vi ".LVLIBP CD XML Updater.vi"(5 "Files Generated by Build":path[](array[path]), 6 "Top Level/Always Included VIs":path[](array[path]), 7 "Destination Path":path, 8 "error in (no error)":errorcluster, 9 "Target Name":string, 10 "Build Specification Name":string, 11 "Project Path":path) -> (0 "error out":errorcluster)   [LabVIEW 2018]
doc: "This VI is called after each run of a build specification. The VI will copy the generated LLB (Engine or System Explorer) into the VeriStand Custom Device folder (...\\Documents\\National Instruments\\NI VeriStand 2013...)."
uses:
  .LVLIBP CD XML Updater/Project XML Editor/Project XML Editor.lvclass/Project XML Editor.ctl
  <vilib>/xml/Close Reference(Node).vi
  .LVLIBP CD XML Updater/.LVLIBP CD XML Updater.lvlib
  .LVLIBP CD XML Updater/LVLIBP Parser/LVLIBP Parser.lvclass
  .LVLIBP CD XML Updater/Project XML Editor/Project XML Editor.lvclass
  <vilib>/xml/NI_XML.lvlib
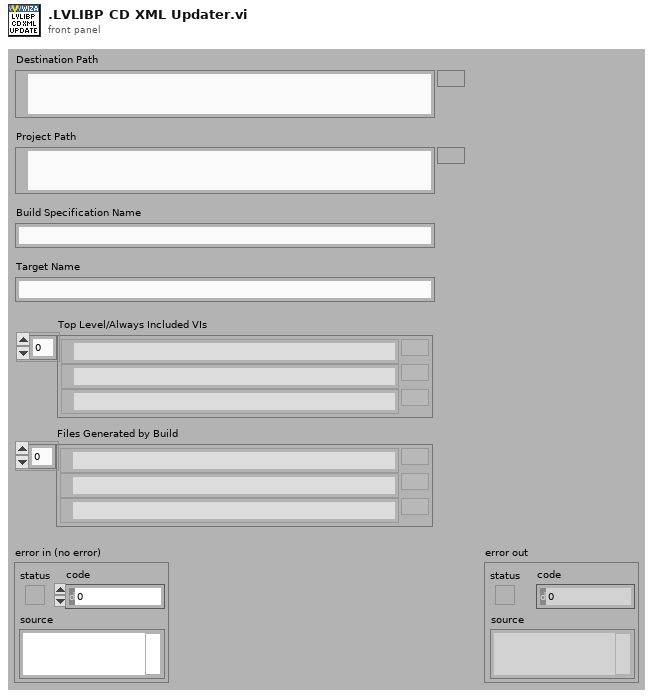
[diagram p1: front panel]
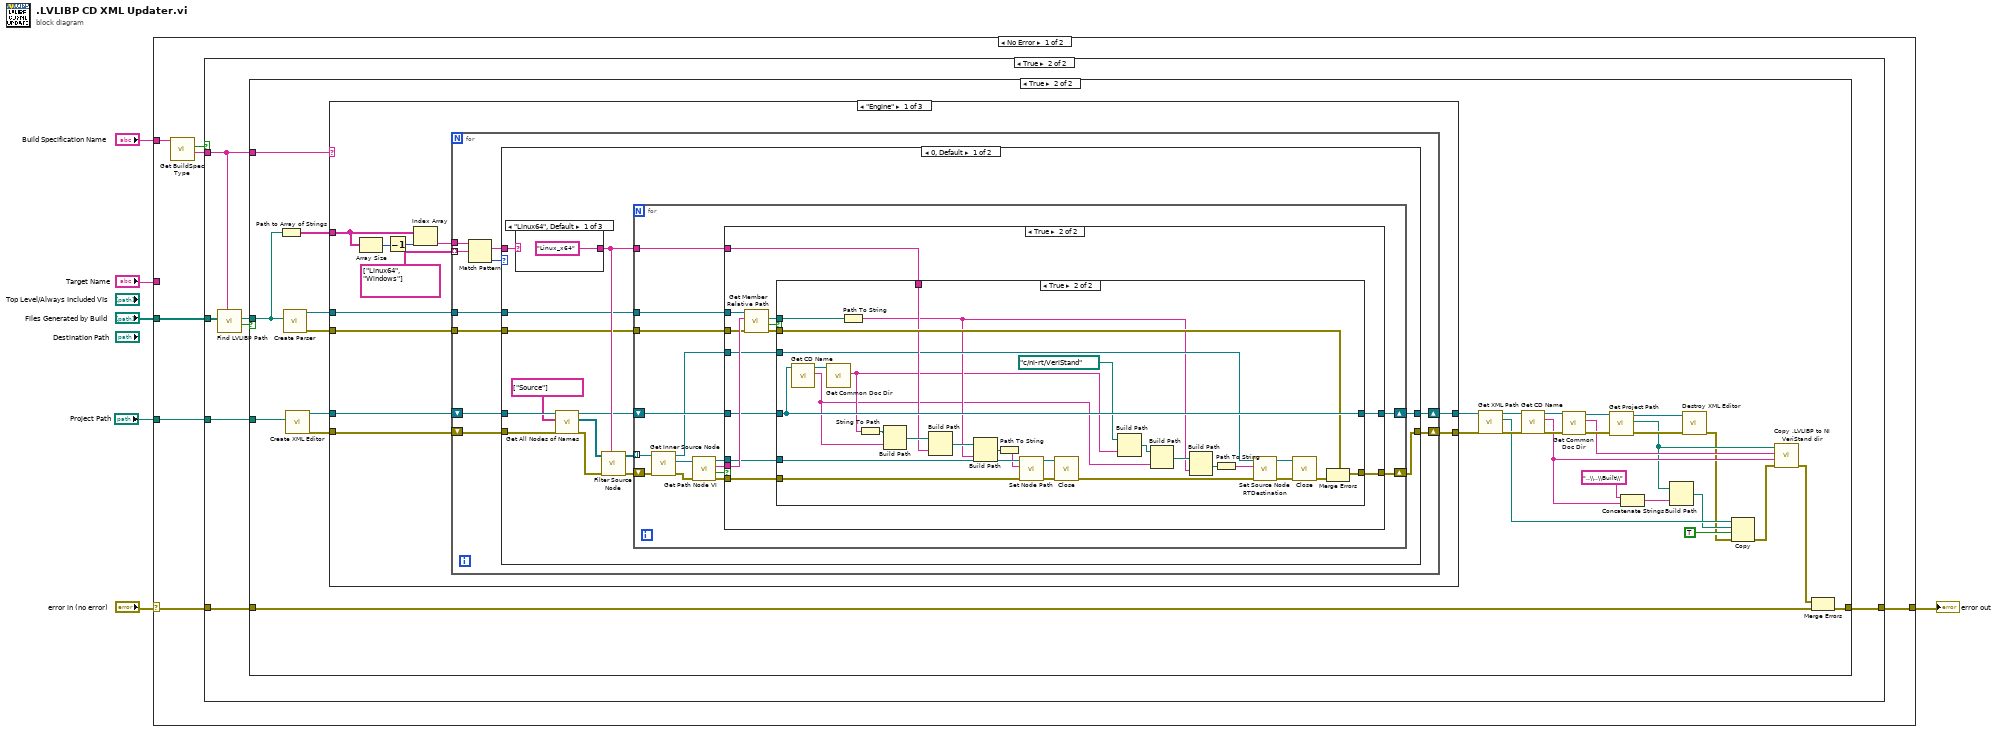
[diagram p0: block diagram]
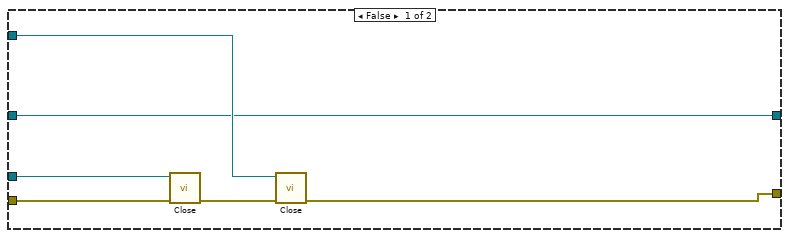
[diagram p5: hidden frame]
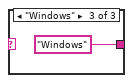
[diagram p7: hidden frame]
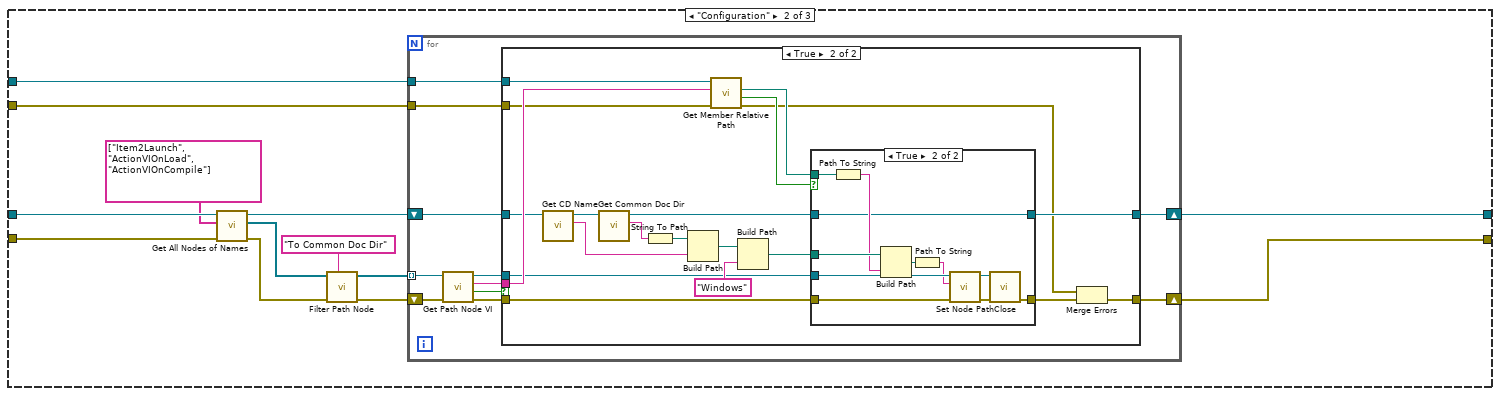
[diagram p9: hidden frame]
diagram:
  n1 = case shown="No Error" "error in (no error)" {
    selector: "error in (no error)" -> [w10 w213]
    tunnel: [w7 w213] -> w4
    tunnel: "Project Path" -> [w9 _]
    tunnel: "Files Generated by Build" -> [w8 _]
    tunnel: "Target Name" -> [_ _]
    tunnel: "Build Specification Name" -> [w13 _]
    frame No Error {
      n2 = call "Get BuildSpec Type.vi"("Build Specification Name in"=w13) -> ("Build Spec Type"=w11:string, "Found ?"=w12:bool)  [unwired: 8 in, 1 out]
      n3 = case shown="True" w12 {
        tunnel: w11 -> [_ w19]
        tunnel: w10 -> [w14 w16]
        tunnel: w9 -> [_ w17]
        tunnel: [w14 w15] -> w7
        tunnel: w8 -> [_ w18]
        frame False {
        }
        frame True {
          n4 = call "Find LVLIBP Path.vi"("Build Type"=w19, "Files Generated by Build"=w18) -> ("Found ?"=w20:bool, "Packed Library Path"=w21:path)  [unwired: 8 in]
          n5 = case shown="True" w20 {
            tunnel: w21 -> [_ w24]
            tunnel: w19 -> [_ w44]
            tunnel: w17 -> [_ w45]
            tunnel: w16 -> [w22 w38]
            tunnel: [w22 w36] -> w15
            frame False {
            }
            frame True {
              n6 = Path to Array of Strings(0:w24) -> (2:w23:string[])  [unwired: 1 out]
              n7 = call "Create Parser.vi"("LVLIBP Path"=w24) -> ("error out"=w48:errorcluster, "LVLIBP Parser out"=w49:refnum<class "LVLIBP Parser.lvclass">)  [unwired: 9 in]
              n8 = call "Create XML Editor.vi"("XML or Project Path"=w45) -> ("error out"=w47:errorcluster, "Project XML Editor out"=w46:refnum<class "Project XML Editor.lvclass">)  [unwired: 9 in]
              n9 = case shown="\"Engine\"" w44 {
                tunnel: w49 -> [w57 w155 _]
                tunnel: w48 -> [w56 w154 _]
                tunnel: w47 -> [w60 w162 w211]
                tunnel: w46 -> [w59 w164 w212]
                tunnel: [w54 w156 w211] -> w40
                tunnel: [w55 w152 w212] -> w35
                tunnel: w23 -> [w53 _ _]
                frame "Engine" {
                  n10 = Array Size(array=w53) -> (size(s)=w52:i32)
                  n11 = Decrement(x=w52) -> (x-1=w51:i32)
                  n12 = Index Array(array=w53, index=w51) -> (element=w50:string)
                  n13 = for {
                    tunnel: string[] ["Linux64", "Windows"] ("Node Names") -> [w68] mode=indexing
                    tunnel: w57 -> [w65]
                    tunnel: w56 -> [w64]
                    shift-right: [w63] -> w55
                    shift-left: w59 -> [w69]
                    shift-right: [w62] -> w54
                    shift-left: w60 -> [w70]
                    tunnel: w50 -> [w61]
                    n14 = Match Pattern(string=w61, regular expression=w68) -> (match substring=w66:string, offset past match=w67:i32)  [unwired: 1 in, 2 out]
                    n15 = case shown="0, Default" w67 {
                      tunnel: w70 -> [w84 w150]
                      tunnel: w69 -> [w83 w151]
                      tunnel: w66 -> [w79 _]
                      tunnel: w65 -> [w75 _]
                      tunnel: w64 -> [w74 _]
                      tunnel: [w72 w151] -> w63
                      tunnel: [w71 w150] -> w62
                      frame 0, Default {
                        n16 = case shown="\"Linux64\", Default" w79 {
                          tunnel: ["Linux_x64" _ "Windows"] -> w76
                          frame "Linux64", Default {
                          }
                          frame "None" {
                          }
                          frame "Windows" {
                          }
                        }
                        n17 = call "Get All Nodes of Names.vi"("error in (no error)"=w84, "Node Names"=string[] ["Source"], "Project XML Editor in"=w83) -> ("error out"=w80:errorcluster, "Nodes Array out"=w81:refnum<k20>[], "Project XML Editor out"=w73:refnum<class "Project XML Editor.lvclass">)  [unwired: 6 in]
                        n18 = call "Filter Source Node.vi"("Supported Target Type"=w76, "error in"=w80, "Nodes Array in"=w81) -> ("error out"=w77:errorcluster, "Nodes Array out"=w78:refnum<k20>[])  [unwired: 7 in]
                        n19 = for {
                          tunnel: w78 -> [w98] mode=indexing
                          tunnel: w76 -> [w88]
                          tunnel: w75 -> [w90]
                          tunnel: w74 -> [w89]
                          shift-right: [w87] -> w72
                          shift-left: w73 -> [w91]
                          shift-right: [w86] -> w71
                          shift-left: w77 -> [w99]
                          n20 = call "Get Inner Source Node.vi"("error in (no error)"=w99, "Node ref in"=w98) -> ("error out"=w96:errorcluster, "Inner Source Node"=w97:refnum<k20>, "Node ref out"=w85:refnum<k20>)  [unwired: 6 in, 1 out]
                          n21 = call "Get Path Node VI.vi"("error in (no error)"=w96, "Node ref in"=w97) -> ("error out"=w95:errorcluster, "Found ?"=w94:bool, "VI Name out"=w93:string, "Node ref out"=w92:refnum<k20>)  [unwired: 6 in]
                          n22 = case shown="True" w94 {
                            tunnel: w93 -> [_ w113]
                            tunnel: w91 -> [w101 w103]
                            tunnel: w92 -> [_ w111]
                            tunnel: w95 -> [w100 w110]
                            tunnel: [w100 w108] -> w86
                            tunnel: [w101 w103] -> w87
                            tunnel: w90 -> [_ w107]
                            tunnel: w89 -> [_ w106]
                            tunnel: w88 -> [_ w105]
                            tunnel: w85 -> [_ w104]
                            frame False {
                            }
                            frame True {
                              n23 = call "Get Member Relative Path.vi"("error in (no error)"=w106, "Member Name"=w113, "LVLIBP Parser in"=w107) -> ("error out"=w109:errorcluster, "Found ?"=w102:bool, "Path"=w112:path)  [unwired: 5 in, 1 out]
                              n24 = case shown="True" w102 {
                                tunnel: w112 -> [_ w145]
                                tunnel: w111 -> [w119 w143]
                                tunnel: w110 -> [w118 w142]
                                tunnel: w109 -> [_ w140]
                                tunnel: [w114 w139] -> w108
                                tunnel: w105 -> [_ w138]
                                tunnel: w104 -> [w117 w137]
                                tunnel: w103 -> [w115 w120]
                                tunnel: [w115 w120] -> _
                                frame False {
                                n25 = call-poly <vilib>:"Close.vi"("error in (no error)"=w118, "node"=w119) -> ("error out"=w116:errorcluster)  [unwired: 7 in]
                                n26 = call-poly <vilib>:"Close.vi"("error in (no error)"=w116, "node"=w117) -> ("error out"=w114:errorcluster)  [unwired: 7 in]
                                }
                                frame True {
                                n27 = call "Get CD Name.vi"("Project XML Editor in"=w120) -> ("CD Name"=w125:string, "Project XML Editor out"=w141:refnum<class "Project XML Editor.lvclass">)  [unwired: 9 in]
                                n28 = call "Get Common Doc Dir.vi"("Project XML Editor in"=w141) -> ("Common Doc Dir"=w126:string)  [unwired: 9 in, 1 out]
                                n29 = Path To String(path=w145) -> (string=w128:string)
                                n30 = String To Path(string=w126) -> (path=w147:path)
                                n31 = Build Path(base path=w147, name or relative path=w125) -> (appended path=w146:path)
                                n32 = Build Path(base path=w146, name or relative path=w138) -> (appended path=w144:path)
                                n33 = Build Path(base path=w144, name or relative path=w128) -> (appended path=w132:path)
                                n34 = Path To String(path=w132) -> (string=w131:string)
                                n35 = call "Set Node Path.vi"("error in (no error)"=w142, "Path in"=w131, "Node ref in"=w143) -> ("error out"=w130:errorcluster, "Node ref out"=w129:refnum<k20>)  [unwired: 6 in, 1 out]
                                n36 = call-poly <vilib>:"Close.vi"("error in (no error)"=w130, "node"=w129) -> ("error out"=w136:errorcluster)  [unwired: 7 in]
                                n37 = Build Path(base path=path "c:/ni-rt/VeriStand", name or relative path=w126) -> (appended path=w134:path)
                                n38 = Build Path(base path=w134, name or relative path=w125) -> (appended path=w133:path)
                                n39 = Build Path(base path=w133, name or relative path=w128) -> (appended path=w127:path)
                                n40 = Path To String(path=w127) -> (string=w124:string)
                                n41 = call "Set Source Node RTDestination.vi"("error in (no error)"=w136, "Path in"=w124, "Node ref in"=w137) -> ("error out"=w123:errorcluster, "Node ref out"=w122:refnum<k20>)  [unwired: 6 in, 1 out]
                                n42 = call-poly <vilib>:"Close.vi"("error in (no error)"=w123, "node"=w122) -> ("error out"=w121:errorcluster)  [unwired: 7 in]
                                n43 = Merge Errors(w140, w121) -> (w139:errorcluster)
                                }
                              }
                            }
                          }
                        }
                      }
                      frame -1 {
                      }
                    }
                  }
                }
                frame "Configuration" {
                  n44 = call "Get All Nodes of Names.vi"("error in (no error)"=w162, "Node Names"=string[] ["Item2Launch", "ActionVIOnLoad", "ActionVIOnCompile"], "Project XML Editor in"=w164) -> ("error out"=w161:errorcluster, "Nodes Array out"=w160:refnum<k20>[], "Project XML Editor out"=w153:refnum<class "Project XML Editor.lvclass">)  [unwired: 6 in]
                  n45 = call "Filter Path Node.vi"("Node Path Type"="To Common Doc Dir" ("y"), "error in"=w161, "Nodes Array in"=w160) -> ("error out"=w157:errorcluster, "Nodes Array out"=w158:refnum<k20>[])  [unwired: 7 in]
                  n46 = for {
                    tunnel: w158 -> [w175] mode=indexing
                    shift-right: [w168] -> w156
                    shift-left: w157 -> [w174]
                    tunnel: w154 -> [w165]
                    shift-right: [w166] -> w152
                    shift-left: w153 -> [w171]
                    tunnel: w155 -> [w173]
                    n47 = call "Get Path Node VI.vi"("error in (no error)"=w174, "Node ref in"=w175) -> ("error out"=w169:errorcluster, "Found ?"=w167:bool, "VI Name out"=w172:string, "Node ref out"=w170:refnum<k20>)  [unwired: 6 in]
                    n48 = case shown="True" w167 {
                      tunnel: w173 -> [_ w197]
                      tunnel: w172 -> [_ w196]
                      tunnel: w171 -> [w177 w186]
                      tunnel: w170 -> [_ w188]
                      tunnel: w169 -> [w176 w187]
                      tunnel: [w176 w178] -> w168
                      tunnel: [w177 w181] -> w166
                      tunnel: w165 -> [_ w183]
                      frame False {
                      }
                      frame True {
                        n49 = call "Get CD Name.vi"("Project XML Editor in"=w186) -> ("CD Name"=w184:string, "Project XML Editor out"=w185:refnum<class "Project XML Editor.lvclass">)  [unwired: 9 in]
                        n50 = call "Get Common Doc Dir.vi"("Project XML Editor in"=w185) -> ("Common Doc Dir"=w195:string, "Project XML Editor out"=w182:refnum<class "Project XML Editor.lvclass">)  [unwired: 9 in]
                        n51 = String To Path(string=w195) -> (path=w194:path)
                        n52 = Build Path(base path=w194, name or relative path=w184) -> (appended path=w193:path)
                        n53 = call "Get Member Relative Path.vi"("error in (no error)"=w183, "Member Name"=w196, "LVLIBP Parser in"=w197) -> ("error out"=w179:errorcluster, "Found ?"=w191:bool, "Path"=w190:path)  [unwired: 5 in, 1 out]
                        n54 = Build Path(base path=w193, name or relative path="Windows") -> (appended path=w189:path)
                        n55 = case shown="True" w191 {
                          tunnel: w190 -> [_ w210]
                          tunnel: w189 -> [_ w209]
                          tunnel: w188 -> [_ w207]
                          tunnel: w187 -> [w199 w204]
                          tunnel: [w199 w200] -> w180
                          tunnel: w182 -> [w198 w203]
                          tunnel: [w198 w203] -> w181
                          frame False {
                          }
                          frame True {
                            n56 = Path To String(path=w210) -> (string=w208:string)
                            n57 = Build Path(base path=w209, name or relative path=w208) -> (appended path=w206:path)
                            n58 = Path To String(path=w206) -> (string=w205:string)
                            n59 = call "Set Node Path.vi"("error in (no error)"=w204, "Path in"=w205, "Node ref in"=w207) -> ("error out"=w202:errorcluster, "Node ref out"=w201:refnum<k20>)  [unwired: 6 in, 1 out]
                            n60 = call-poly <vilib>:"Close.vi"("error in (no error)"=w202, "node"=w201) -> ("error out"=w200:errorcluster)  [unwired: 7 in]
                          }
                        }
                        n61 = Merge Errors(w179, w180) -> (w178:errorcluster)
                      }
                    }
                  }
                }
                frame "None", Default {
                }
              }
              n62 = call "Get XML Path.vi"("Project XML Editor in"=w35) -> ("XML Path"=w30:path, "Project XML Editor out"=w32:refnum<class "Project XML Editor.lvclass">)  [unwired: 9 in]
              n63 = call "Get CD Name.vi"("Project XML Editor in"=w32) -> ("CD Name"=w31:string, "Project XML Editor out"=w43:refnum<class "Project XML Editor.lvclass">)  [unwired: 9 in]
              n64 = call "Get Common Doc Dir.vi"("Project XML Editor in"=w43) -> ("Common Doc Dir"=w39:string, "Project XML Editor out"=w42:refnum<class "Project XML Editor.lvclass">)  [unwired: 9 in]
              n65 = call "Get Project Path.vi"("Project XML Editor in"=w42) -> ("Source Project Path"=w27:path, "Project XML Editor out"=w41:refnum<class "Project XML Editor.lvclass">)  [unwired: 8 in, 1 out]
              n66 = Concatenate Strings("..\\..\\Built\\" ("string"), w31) -> (w33:string)
              n67 = Build Path(base path=w27, name or relative path=w33) -> (appended path=w29:path)
              n68 = call "Destroy XML Editor.vi"("error in (no error)"=w40, "Project XML Editor in"=w41) -> ("error out"=w26:errorcluster)  [unwired: 9 in]
              n69 = Copy(8:w26, 9:TRUE ("overwrite (F)"), 10:w29, 11:w30) -> (0:w25:errorcluster)  [unwired: 1 in, 2 out]
              n70 = call "Copy .LVLIBP to NI VeriStand dir.vi"("error in (no error)"=w25, "CD name"=w31, "CD Folder name"=w39, "Project Path"=w27) -> ("error out"=w37:errorcluster)  [unwired: 7 in]
              n71 = Merge Errors(w37, w38) -> (w36:errorcluster)
            }
          }
        }
      }
    }
    frame Error {
    }
  }
  "error out" <- w4
